vi "工位状态.vi"(7 "枚举":enum16{"Read", "Write"}(ring), 11 "Status_Write":i16) -> (2 "右工位在位":bool, 3 "左工位在位":bool)   [LabVIEW 2020]
uses:
  Libraries/S7/S7.lvlib
panel:
  out "Status_Read":dbl
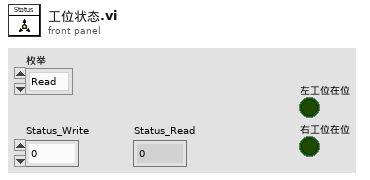
[diagram p1: front panel]
types:
  T1 = typedef "S7.lvlib/Read_Data (Reply Payload)--cluster.ctl" = cluster{"读取成功":bool, "数据":u32[], "Read_Data_error":errorcluster}
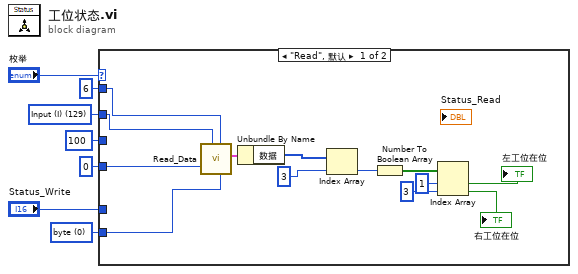
[diagram p0: block diagram]
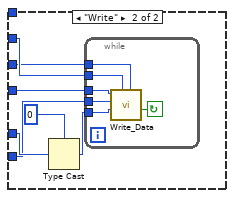
[diagram p2: hidden frame]
diagram:
  w3 = u16 0 items=["byte", "word", "Dword"] ("数据类型")
  w4 = u8 129 items=["I/O (P)"=128, "Input (I)"=129, "Output (Q)"=130, "Bit Memory (M)"=131, "Data (DB)"=132, "Instance Data (DI)"=133, "Local Data (L)"=134, "Predecessor Local Data (VL)"=135] ("寄存器类型")
  n1 = case shown="\"Read\", 默认" "枚举" {
    tunnel: u16 100 ("DB #") -> [_ w22]
    tunnel: u32 0 ("起始地址") -> [w20 w21]
    tunnel: w4 -> [w19 w24]
    tunnel: u16 6 ("读取长度") -> [w18 _]
    tunnel: w3 -> [w17 w23]
    tunnel: "Status_Write" -> [_ w25]
    frame "Read", Default {
      n2 = call "Read_Data.vi"("数据类型"=w17, "读取长度"=w18, "寄存器类型"=w19, "起始地址"=w20) -> ("Reply Payload"=w16:T1)  [unwired: 5 in, 2 out]
      n3 = Unbundle By Name(w16) -> ("数据"=w15:u32[])
      n4 = Index Array(array=w15, index=3 ("索引")) -> (element=w13:u32)
      n5 = Number To Boolean Array(number=w13) -> (Boolean array=w12:bool[])
      n6 = Index Array(array=w12, index #1=1 ("索引"), index #2=3 ("索引")) -> (element #1=→"左工位在位":bool, element #2=→"右工位在位":bool)
    }
    frame "Write" {
      n7 = Type Cast(type=u16 0, x=w25) -> (*(type *) &x=w26:u16)
      n8 = while {
        tunnel: w26 -> [w33]
        tunnel: w24 -> [w32]
        tunnel: w23 -> [w31]
        tunnel: w22 -> [w30]
        tunnel: w21 -> [w29]
        stop <- w28 continue-if-true
        n9 = call "Write_Data.vi"("DB #"=w30, "寄存器类型"=w32, "写入数据"=w33, "数据类型"=w31, "写入地址"=w29) -> ("timed out?"=w28:bool)  [unwired: 4 in, 2 out]
      }
    }
  }
